vi "Durability.vi"(7 "Notifier Data":T1, 8 "error in (no error)":errorcluster, 9 "notifier out":refnum<notifier>, 10 "Step Duration":dbl, 11 "Data Cluster":T3) -> (0 "error out":errorcluster, 2 "Averaged Data Array":dbl[][](array[numeric]), 3 "STOP Out":bool)   [LabVIEW 2026, in "Acquisition.lvlib"]
uses:
  Acquisition.lvlib
  Hardware Configuration.ctl
  controls/Durability Test Conditions.ctl
  controls/NotifierAndDataQueue.ctl
  controls/WaveformChartData.ctl
  controls/TestCaseTimer.vi
  Settings/Settings.lvlib
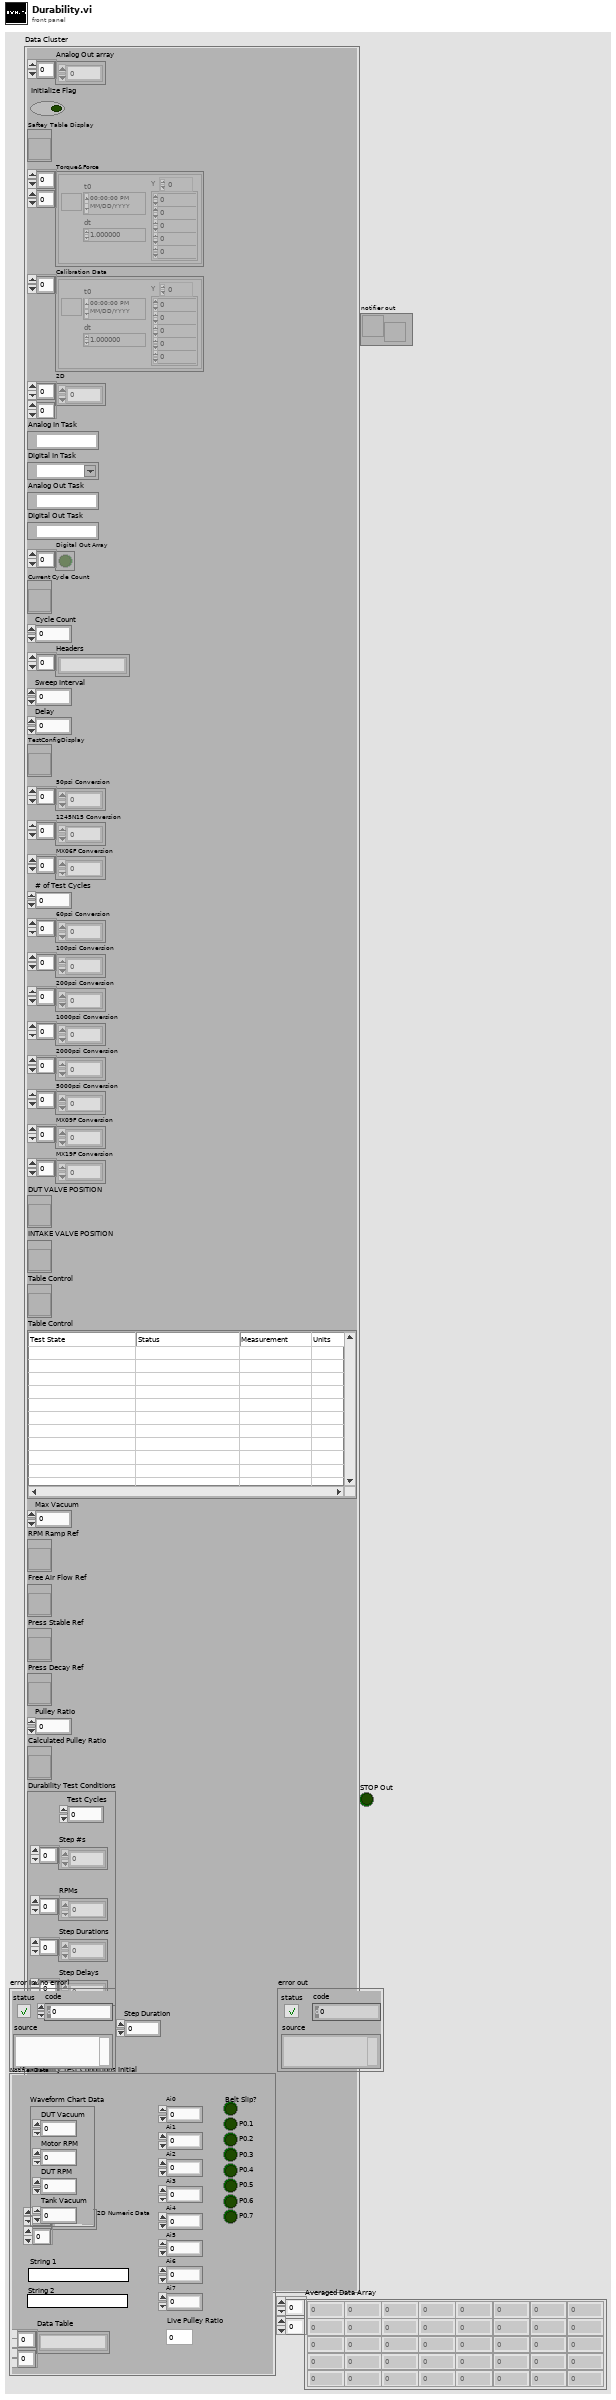
[diagram p1: front panel]
types:
  T1 = typedef "NotifierAndDataQueue.ctl" = cluster{"Ai0":dbl, "Ai1":dbl, "Ai2":dbl, "Ai3":dbl, "Ai4":dbl, "Ai5":dbl, "Ai6":dbl, "Ai7":dbl, "Belt Slip?":bool, "P0.1":bool, "P0.2":bool, "P0.3":bool, "P0.4":bool, "P0.5":bool, "P0.6":bool, "P0.7":bool, "2D Numeric Data":dbl[][], "String 2":string, "String 1":string, "Waveform Chart Data":T2, "Live Pulley Ratio":dbl, "Data Table":string[][]}
  T2 = typedef "Settings.lvlib/WaveformChartData.ctl" = cluster{"DUT Vacuum":dbl, "Motor RPM":dbl, "DUT RPM":dbl, "Tank Vacuum":dbl}
  T3 = typedef "Acquisition.lvlib/Hardware Configuration.ctl" = cluster{"Analog Out array":dbl[], "Initialize Flag":bool, "Saftey Table Display":refnum<vi>, "Torque&Force":waveform(dbl)[][], "Calibration Data":waveform(dbl)[], "2D":dbl[][], "Analog In Task":refnum<k21>, "Digital In Task":refnum<k21>, "Analog Out Task":refnum<k21>, "Digital Out Task":refnum<k21>, "Digital Out Array":bool[], "Current Cycle Count":refnum<vi>, "Cycle Count":u64, "Headers":string[], "Sweep Interval":u64, "Delay":u64, "TestConfigDisplay":refnum<vi>, "50psi Conversion":dbl[], "1245N15 Conversion":dbl[], "MX06F Conversion":dbl[], "# of Test Cycles":u64, "60psi Conversion":dbl[], "100psi Conversion":dbl[], "200psi Conversion":dbl[], "1000psi Conversion":dbl[], "2000psi Conversion":dbl[], "5000psi Conversion":dbl[], "MX09F Conversion":dbl[], "MX19F Conversion":dbl[], "DUT VALVE POSITION":refnum<vi>, "INTAKE VALVE POSITION":refnum<vi>, "Table Control":refnum<vi>, "Table Control":string[][], "Max Vacuum":dbl, "RPM Ramp Ref":refnum<vi>, "Free Air Flow Ref":refnum<vi>, "Press Stable Ref":refnum<vi>, "Press Decay Ref":refnum<vi>, "Pulley Ratio":dbl, "Calculated Pulley Ratio":refnum<vi>, "Durability Test Conditions":T4, "# of Durab Steps":dbl, "manual aquire timer":dbl, "Durability Test Conditions Initial":T4}
  T4 = typedef "Durability Test Conditions.ctl" = cluster{"Step #s":dbl[], "RPMs":dbl[], "Step Durations":dbl[], "Step Delays":dbl[], "Test Cycles":dbl}
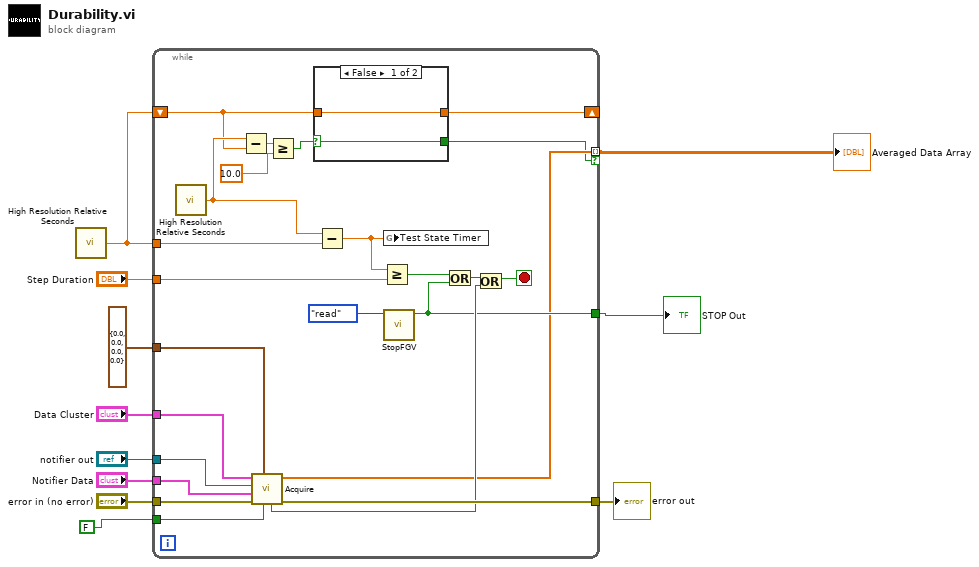
[diagram p0: block diagram]
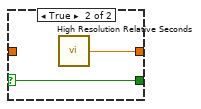
[diagram p2: hidden frame]
diagram:
  n1 = call <vilib>:"High Resolution Relative Seconds.vi"() -> ("relative seconds"=w3:dbl)
  n2 = while {
    tunnel: w3 -> [w19]
    tunnel: "Step Duration" -> [w35]
    tunnel: "error in (no error)" -> [w34]
    tunnel: "notifier out" -> [w33]
    tunnel: "Data Cluster" -> [w32]
    tunnel: "Notifier Data" -> [w31]
    tunnel: T2 {"DUT Vacuum"=0.0, "Motor RPM"=0.0, "DUT RPM"=0.0, "Tank Vacuum"=0.0} ("Waveform Chart Data") -> [w30]
    tunnel: FALSE -> [w27]
    tunnel: [w25] -> w5
    tunnel: [w21] -> w4
    shift-right: [w20] -> _
    shift-left: w3 -> [w12]
    tunnel: [w15] -> w2 mode=indexing if=w14
    stop <- w24 stop-if-true
    n3 = call <vilib>:"High Resolution Relative Seconds.vi"() -> ("relative seconds"=w13:dbl)
    n4 = Subtract(x=w13, y=w12) -> (x-y=w18:dbl)
    n5 = call "Acquire.vi"("Need Belt Monitor?"=w27, "Waveform Chart Data"=w30, "error in (no error)"=w34, "Notifiier Data"=w31, "notifier out"=w33, "Hardware Resources in"=w32) -> ("error out"=w25:errorcluster, "Averaged Data Array"=w15:dbl[], "Belt Slip?"=w22:bool)  [unwired: 1 in, 2 out]
    n6 = Greater Or Equal?(x=w18, y=10.0) -> (x >= y?=w17:bool)
    n7 = case shown="False" w17 {
      selector: w17 -> [w36 w38]
      tunnel: [w37 w39] -> w20
      tunnel: w12 -> [w37 _]
      tunnel: [w36 w38] -> w14
      frame False {
      }
      frame True {
        n8 = call <vilib>:"High Resolution Relative Seconds.vi"() -> ("relative seconds"=w39:dbl)
      }
    }
    n9 = Subtract(x=w13, y=w19) -> (x-y=w26:dbl)
    n10 = Greater Or Equal?(x=w26, y=w35) -> (x >= y?=w28:bool)
    n11 = global write "TestCaseTimer.vi" "Test State Timer"(w26) -> ()
    n12 = call "StopFGV.vi"("Enum"=enum16{"init", "write", "read"}."read") -> ("STOP Out"=w21:bool)  [unwired: 9 in, 1 out]
    n13 = Or(x=w28, y=w21) -> (x .or. y?=w23:bool)
    n14 = Or(x=w23, y=w22) -> (x .or. y?=w24:bool)
  }
  "error out" <- w5
  "STOP Out" <- w4
  "Averaged Data Array" <- w2
